vi "CMD_SETERRORMODE.vi"(8 "error in (no error)":errorcluster, 10 "Arguments":string[](array[string]), 11 "gScript Interpreter in":refnum<class "gScript Interpreter.lvclass">) -> (0 "error out":errorcluster, 3 "gScript Interpreter out":refnum<class "gScript Interpreter.lvclass">)   [LabVIEW 2017, in "gScript Interpreter.lvclass"]
uses:
  gScript Interpreter.lvclass
  Type Definitions/Error Mode.ctl
  gScript Interpreter.lvclass/gScript Interpreter.ctl
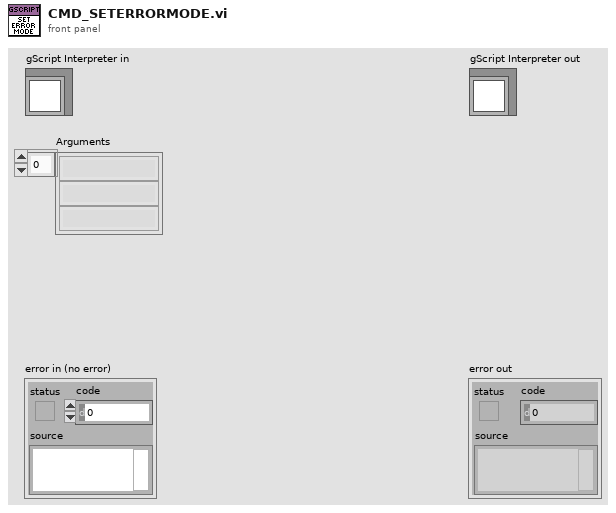
[diagram p1: front panel]
types:
  T1 = typedef "Error Mode.ctl" = enum16{"default", "prompt", "setvar"}
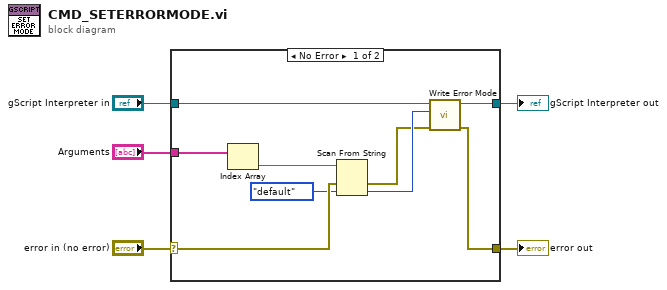
[diagram p0: block diagram]
diagram:
  n1 = case shown="No Error" "error in (no error)" {
    selector: "error in (no error)" -> [w12 w16]
    tunnel: [w6 w16] -> w4
    tunnel: [w7 w15] -> w2
    tunnel: "gScript Interpreter in" -> [w8 w15]
    tunnel: "Arguments" -> [w14 _]
    frame No Error {
      n2 = Index Array(array=w14) -> (element=w13:string)  [unwired: 1 in]
      n3 = Scan From String(input string=w13, error in=w12, default 1=Error_Mode."default" ("Error Mode")) -> (error out=w9:errorcluster, output 1=w10:T1)  [unwired: 2 in, 2 out]
      n4 = call "Write Error Mode.vi"("error in (no error)"=w9, "Error Mode"=w10, "gScript Interpreter in"=w8) -> ("error out"=w6:errorcluster, "gScript Interpreter out"=w7:refnum<class "gScript Interpreter.lvclass">)  [unwired: 7 in]
    }
    frame Error {
    }
  }
  "error out" <- w4
  "gScript Interpreter out" <- w2
